vi "Search_and_match.vi"(0 "Learn Mode":u32(ring)=1 items=["All", "Shift Information", "Rotation Information"], 1 "Feature Mode":u32(ring) items=["Color and Shape", "Color", "Shape "], 2 "Minimum Match Score":sgl=800.0 min=0 max=1000 format="%.2f", 3 "Number of Matches Requested":i32=1 min=1, 4 "Match Mode":u32(ring) items=["Shift Invariant", "Rotation Invariant"], 6 "Ref path":path, 7 "Match Feature Mode":u32(ring) items=["Color and Shape", "Color", "Shape"], 8 "Main Path":path) -> (14 "Number of Matches":i32)   [LabVIEW 2025]
uses:
  <vilib>/vision/NI_Vision_Development_Module.lvlib
panel:
  out "Number of Particles 2":i32
  out "Histogram Report":T1 {"Standard  Variation" format="%.2f"; "Mean Value" format="%.2f"; "Interval Width" format="%.2f"; "Starting Value" format="%.2f"; "Maximal Value" format="%.2f"; "Minimal Value" format="%.2f"}
  in  "Interval Range":cluster{"Minimum":sgl, "Maximum":sgl} {"Maximum" format="%.2f"; "Minimum" format="%.2f"}
  out "error out":errorcluster
  out "Extraced_Image":T2(plugin-control)
  in  "Rotation Angle Ranges (degrees)":cluster{sgl, sgl}[](array[cluster]) {"?" format="%.2f"; "?" format="%.2f"}
  out "Main Image":T2(plugin-control)
  out "Ref image":T2(plugin-control)
  out "Matches":T3(array[cluster]) {"Bounding Box"."y" format="%.2f"; "Bounding Box"."x" format="%.2f"; "Position"."y" format="%.2f"; "Position"."x" format="%.2f"; "Score" format="%.2f"; "Scale" format="%.2f"; "Angle" format="%.2f"}
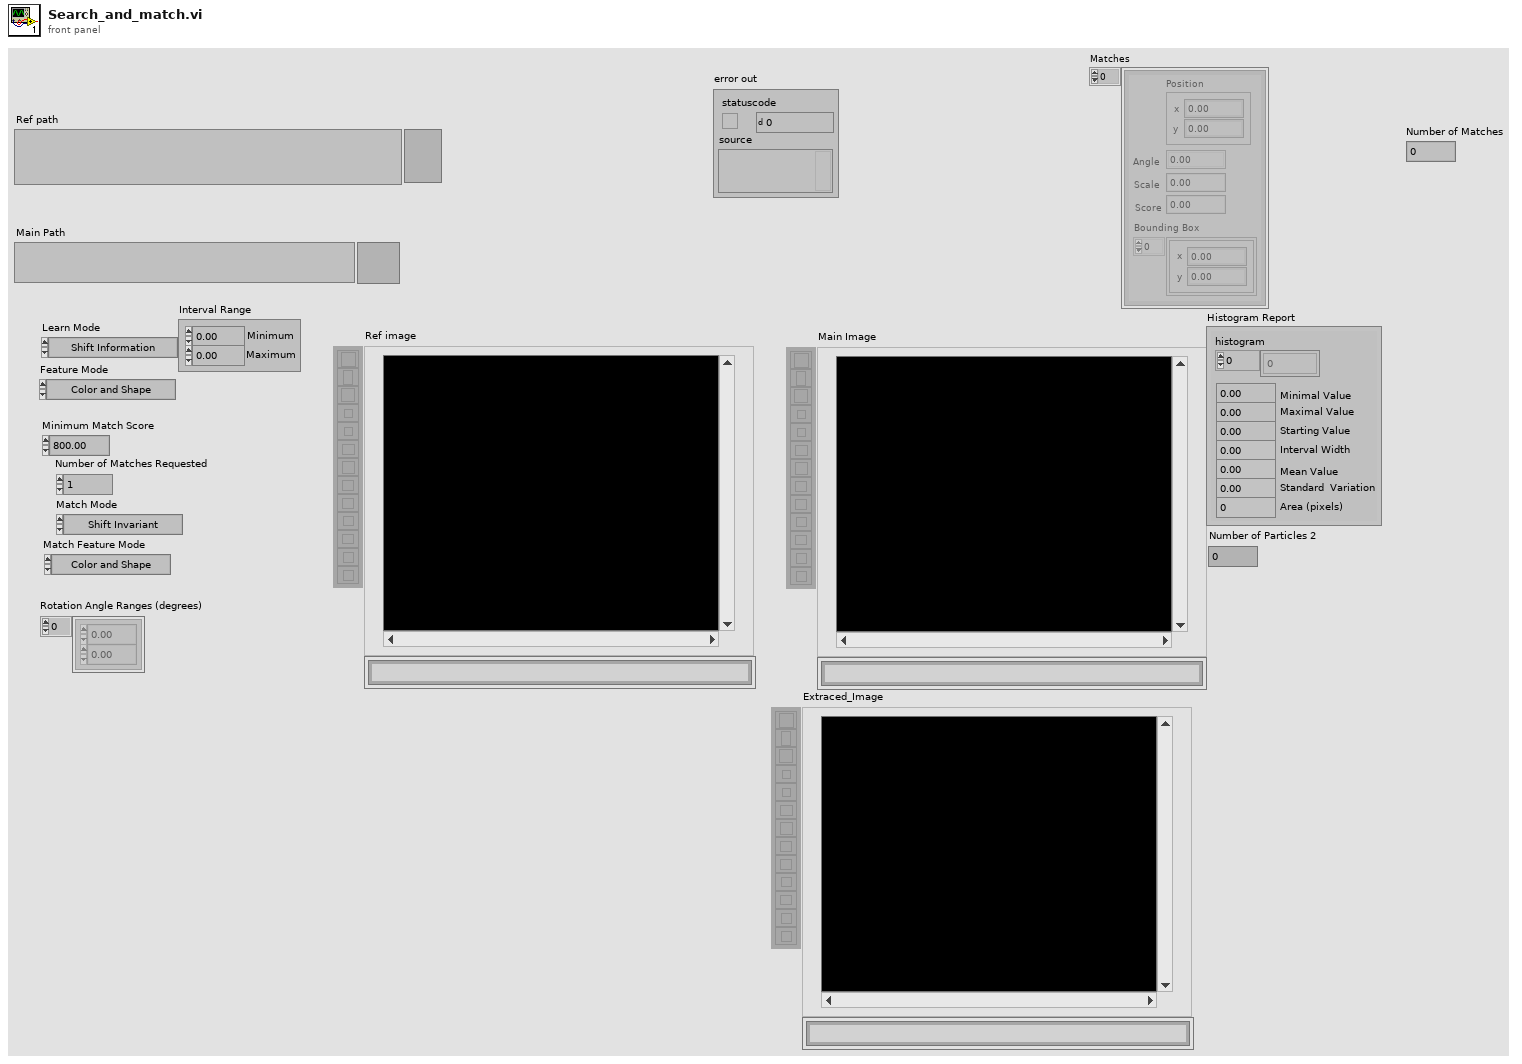
[diagram p1: front panel]
types:
  T1 = cluster{"histogram":u32[], "Minimal Value":sgl, "Maximal Value":sgl, "Starting Value":sgl, "Interval Width":sgl, "Mean Value":sgl, "Standard  Variation":sgl, "Area (pixels)":i32}
  T2 = typedef "IMAQ Image.ctl" = refnum<image>
  T3 = cluster{"Position":cluster{"x":sgl, "y":sgl}, "Angle":sgl, "Scale":sgl, "Score":sgl, "Bounding Box":cluster{"x":sgl, "y":sgl}[]}[]
  T4 = typedef "Image Type" = u32
  T5 = typedef "IMAQ Rectangle" = cluster{"Left":i32, "Top":i32, "Right":i32, "Bottom":i32, "Rotation":dbl}
  T6 = typedef "ROI Descriptor" = cluster{"Global Rectangle":i32[], "Contours":cluster{"ID":enum32{"External", "Internal"}, "Type":u32, "Coordinates":i32[]}[]}
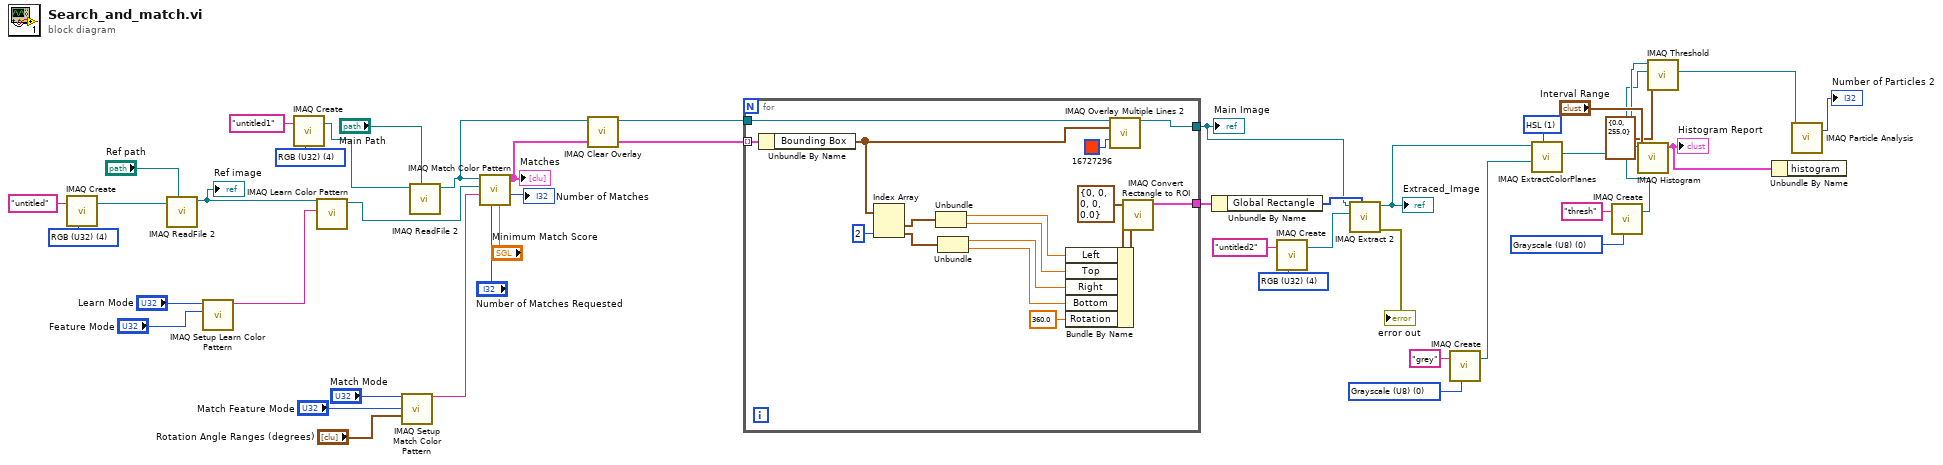
[diagram p0: block diagram]
diagram:
  w4 = T4 0 items=["Grayscale (U8)", "Grayscale (I16)", "Grayscale (SGL)", "Complex (CSG)", "RGB (U32)", "HSL (U32)", "RGB (U64)", "Grayscale (U16)"] ("Image Type")
  w7 = T4 0 items=["Grayscale (U8)", "Grayscale (I16)", "Grayscale (SGL)", "Complex (CSG)", "RGB (U32)", "HSL (U32)", "RGB (U64)", "Grayscale (U16)"] ("Image Type")
  w14 = u16 1 items=["RGB", "HSL", "HSV", "HSI"] ("Color Mode")
  w21 = T4 4 items=["Grayscale (U8)", "Grayscale (I16)", "Grayscale (SGL)", "Complex (CSG)", "RGB (U32)", "HSL (U32)", "RGB (U64)", "Grayscale (U16)"] ("Image Type")
  w40 = T4 4 items=["Grayscale (U8)", "Grayscale (I16)", "Grayscale (SGL)", "Complex (CSG)", "RGB (U32)", "HSL (U32)", "RGB (U64)", "Grayscale (U16)"] ("Image Type")
  w43 = T4 4 items=["Grayscale (U8)", "Grayscale (I16)", "Grayscale (SGL)", "Complex (CSG)", "RGB (U32)", "HSL (U32)", "RGB (U64)", "Grayscale (U16)"] ("Image Type")
  n1 = call "IMAQ Create"("Image Name"="untitled", "Image Type"=w43) -> ("New Image"=w42:T2)  [unwired: 3 in, 1 out]
  n2 = call "IMAQ ReadFile 2"("File Path"="Ref path", "Image"=w42) -> ("Image Out"=w26:T2)  [unwired: 5 in, 4 out]
  "Ref image" <- w26
  n3 = call "IMAQ Setup Learn Color Pattern"("Feature Mode"="Feature Mode", "Learn Mode"="Learn Mode") -> ("Learn Color Pattern Setup Data"=w36:string)  [unwired: 8 in, 1 out]
  n4 = call "IMAQ Create"("Image Name"="untitled1", "Image Type"=w40) -> ("New Image"=w34:T2)  [unwired: 3 in, 1 out]
  n5 = call "IMAQ Learn Color Pattern"("Learn Color Pattern Setup Data"=w36, "Image"=w26) -> ("Template Image Out"=w33:T2)  [unwired: 8 in, 1 out]
  n6 = call "IMAQ Setup Match Color Pattern"("Match Mode"="Match Mode", "Match Feature Mode"="Match Feature Mode", "Rotation Angle Ranges (degrees)"="Rotation Angle Ranges (degrees)") -> ("Match Color Pattern Setup Data"=w32:string)  [unwired: 11 in, 1 out]
  n7 = call "IMAQ ReadFile 2"("File Path"="Main Path", "Image"=w34) -> ("Image Out"=w24:T2)  [unwired: 5 in, 4 out]
  n8 = call "IMAQ Match Color Pattern"("Minimum Match Score"="Minimum Match Score", "Number of Matches Requested"="Number of Matches Requested", "Match Color Pattern Setup Data"=w32, "Template Image"=w33, "Image"=w24) -> ("Number of Matches"=→"Number of Matches":i32, "Matches"=w23:T3)  [unwired: 4 in, 1 out]
  "Matches" <- w23
  n9 = call "IMAQ Clear Overlay"("Image"=w24) -> ("Image Out"=w22:T2)  [unwired: 9 in, 1 out]
  n10 = for {
    tunnel: w22 -> [w60]
    tunnel: w23 -> [w58] mode=indexing
    tunnel: [w57] -> w16
    tunnel: [w46] -> w18
    n11 = Unbundle By Name(w58) -> ("Bounding Box"=w53:cluster{"x":sgl, "y":sgl}[])
    n12 = Index Array(array=w53, index #2=2 ("index")) -> (element #1=w52:cluster{"x":sgl, "y":sgl}, element #2=w51:cluster{"x":sgl, "y":sgl})  [unwired: 1 in]
    n13 = Unbundle(w52) -> ("x"=w50:sgl, "y"=w49:sgl)
    n14 = Unbundle(w51) -> ("x"=w48:sgl, "y"=w47:sgl)
    n15 = Bundle By Name(cluster=T5 {"Left"=0, "Top"=0, "Right"=0, "Bottom"=0, "Rotation"=0.0} ("Rectangle"), "Left"=w50, "Top"=w49, "Right"=w48, "Bottom"=w47, "Rotation"=360.0) -> (w55:T5)
    n16 = call "IMAQ Overlay Multiple Lines 2"("Image"=w60, "Line End Points"=w53, "Color"=u32 16727296) -> ("Image Out"=w57:T2)  [unwired: 11 in, 1 out]
    n17 = call "IMAQ Convert Rectangle to ROI"("Rectangle"=w55) -> ("ROI Descriptor"=w46:T6)  [unwired: 8 in, 1 out]
  }
  "Main Image" <- w16
  n18 = Unbundle By Name(w18) -> ("Global Rectangle"=w17:i32[])
  n19 = call "IMAQ Create"("Image Name"="untitled2", "Image Type"=w21) -> ("New Image"=w19:T2)  [unwired: 3 in, 1 out]
  n20 = call "IMAQ Extract 2"("Optional Rectangle"=w17, "Image Dst"=w19, "Image Src"=w16) -> ("error out"=→"error out":errorcluster, "Image Dst Out"=w5:T2)  [unwired: 7 in]
  "Extraced_Image" <- w5
  n21 = call "IMAQ Create"("Image Name"="grey", "Image Type"=w4) -> ("New Image"=w2:T2)  [unwired: 3 in, 1 out]
  n22 = call "IMAQ ExtractColorPlanes"("Color Mode"=w14, "Green or Sat Plane"=w2, "Image Src"=w5) -> ("Green or Sat Plane out"=w9:T2)  [unwired: 5 in, 3 out]
  n23 = call "IMAQ Create"("Image Name"="thresh", "Image Type"=w7) -> ("New Image"=w6:T2)  [unwired: 3 in, 1 out]
  n24 = call "IMAQ Histogram"("Interval Range"="Interval Range", "Image"=w9) -> ("Histogram Report"=w12:T1)  [unwired: 8 in, 1 out]
  "Histogram Report" <- w12
  n25 = call "IMAQ Threshold"("Range"=cluster{"Lower value":sgl, "Upper value":sgl} {"Lower value"=0.0, "Upper value"=255.0}, "Image Dst"=w6, "Image Src"=w9) -> ("Image Dst Out"=w10:T2)  [unwired: 7 in, 1 out]
  n26 = Unbundle By Name(w12) -> ()  [unwired: 1 out]
  n27 = call "IMAQ Particle Analysis"("Image"=w10) -> ("Number of Particles"=→"Number of Particles 2":i32)  [unwired: 5 in, 5 out]
